vi "GEA3 HEWH Mixing Valve ERD List.vi"(8 "error in (no error)":errorcluster, 11 "Enable Electronic Mixing Valve (EMV) List":bool) -> (0 "error out":errorcluster, 2 "Headers":string[](array[string]), 3 "Read ERD List":T1[](array[typedef]) {"ERD Number" format="%.0x"})   [LabVIEW 2020]
uses:
  type defs/ERD Read Data In.ctl
  type defs/Data Type.ctl
  <vilib>/Utility/error.llb/whitespace.ctl
  library/GEA2_Toolkit.lvlib
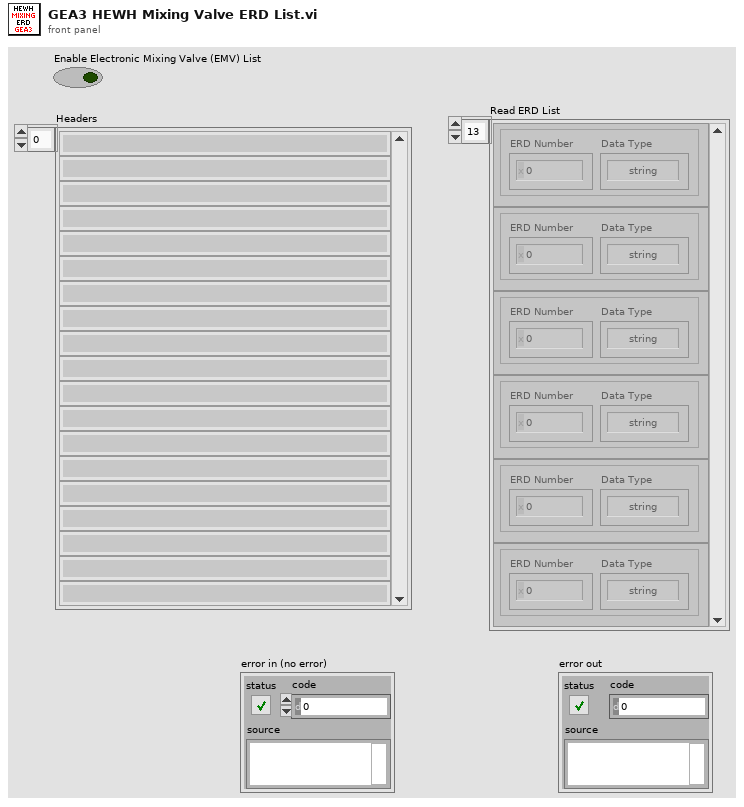
[diagram p1: front panel]
types:
  T1 = typedef "GEA2_Toolkit.lvlib/ERD Read Data In.ctl" = cluster{"ERD Number":u16, "Data Type":T2}
  T2 = typedef "GEA2_Toolkit.lvlib/Data Type.ctl" = enum16{"string", "boolean", "uint8_t", "uint16_t", "uint32_t", "uint64_t", "int8_t", "int16_t", "int32_t", "int64_t"}
  T3 = typedef "whitespace.ctl" = u16
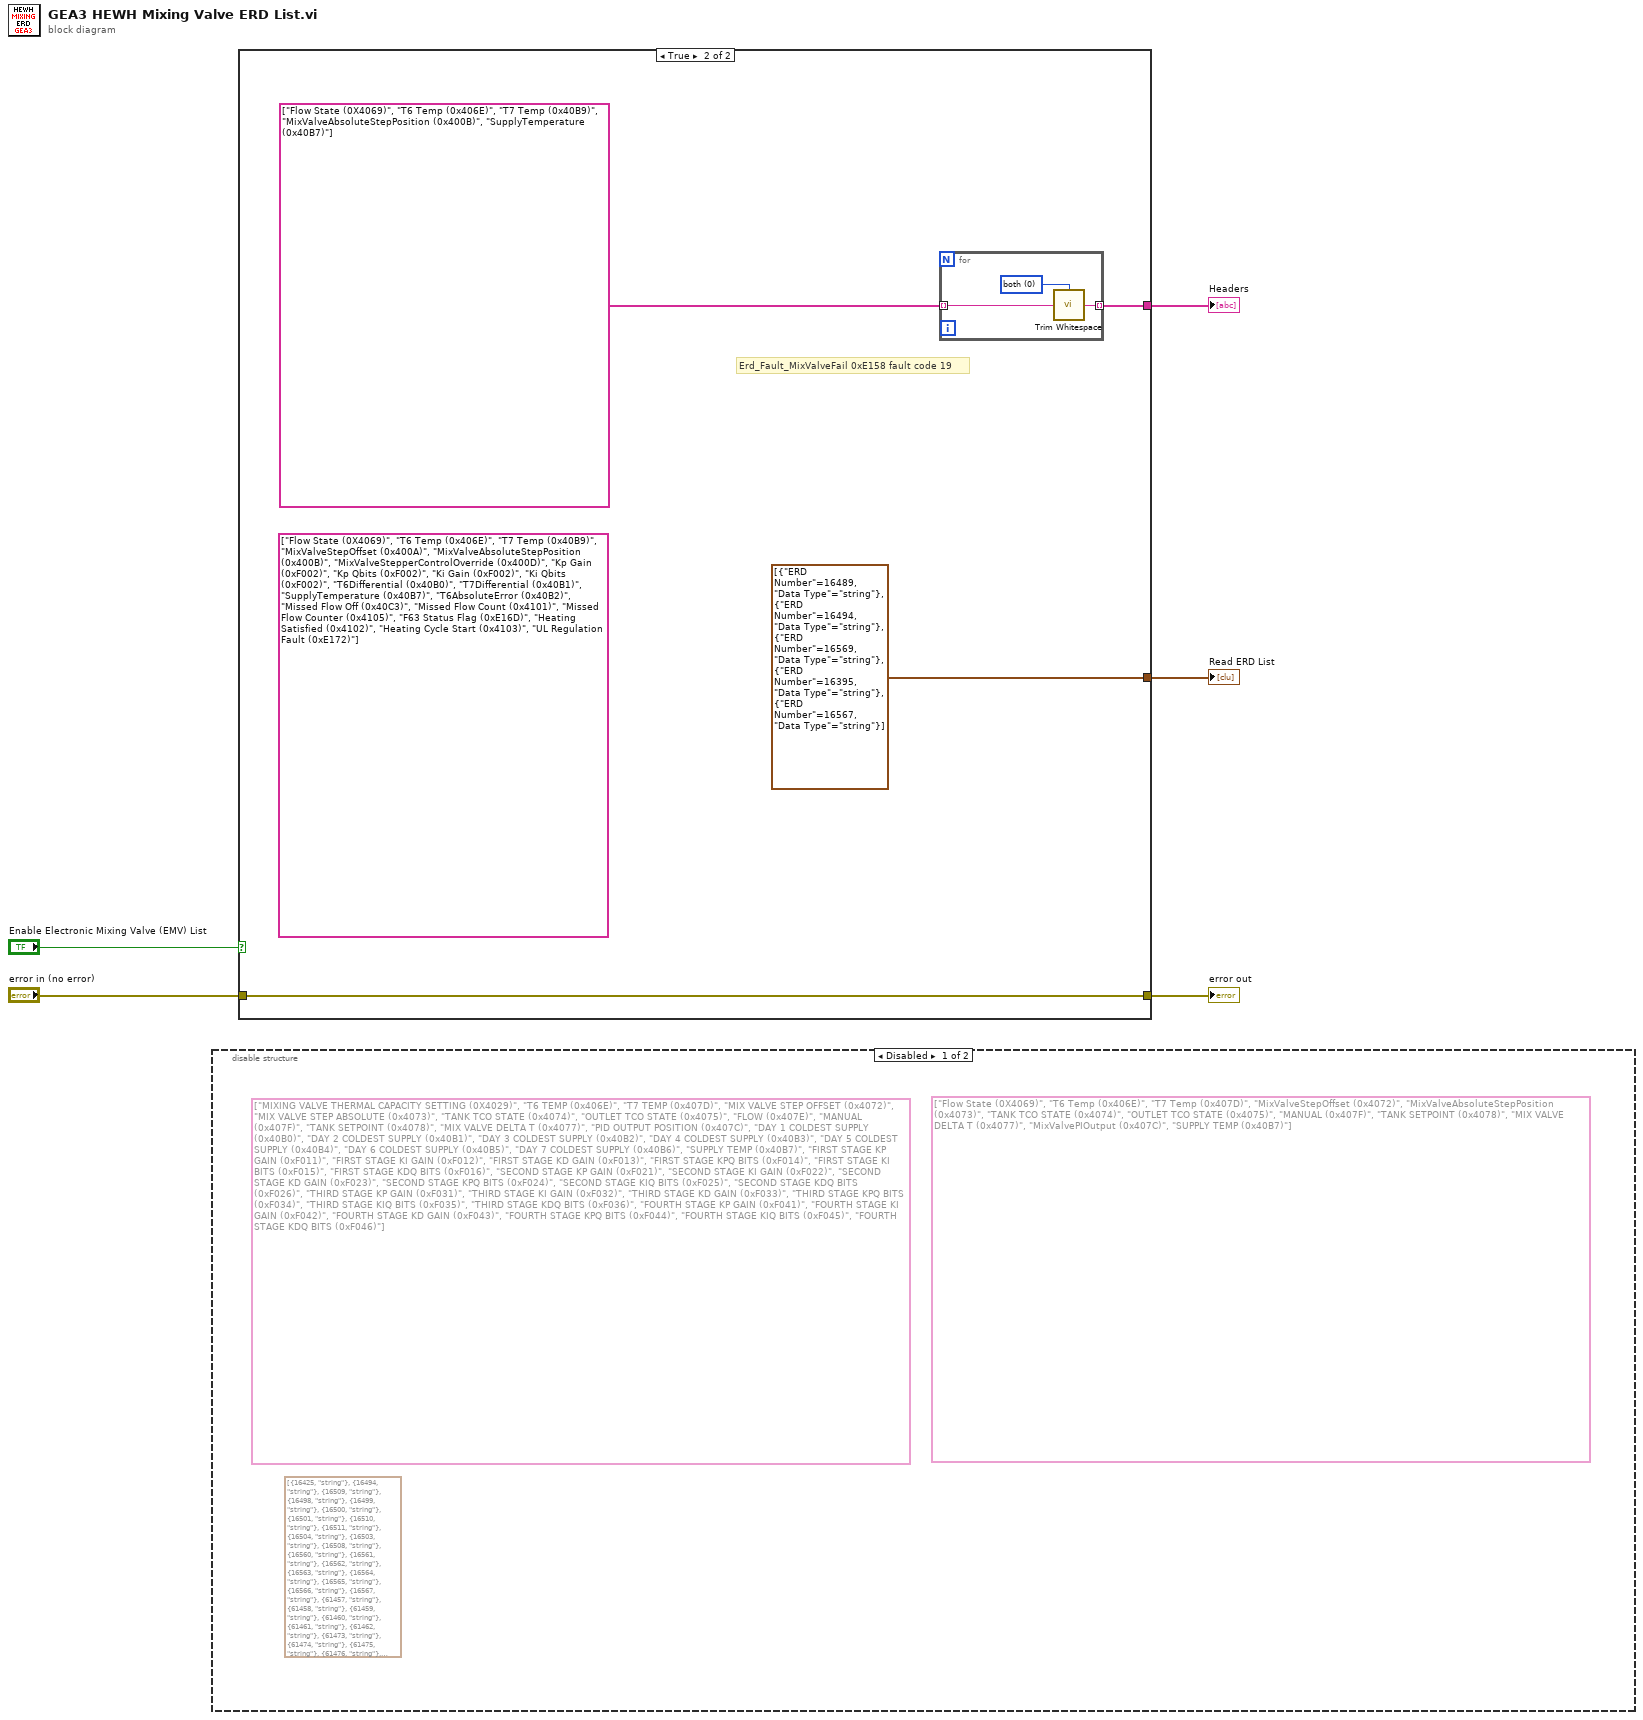
[diagram p0: block diagram]
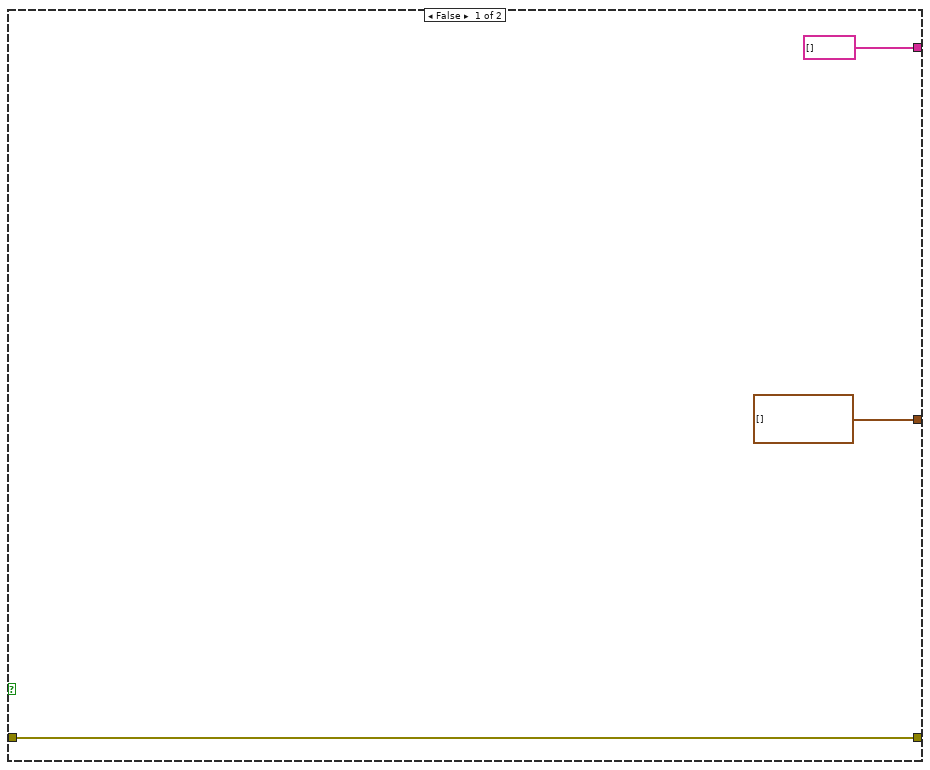
[diagram p3: hidden frame]
diagram:
  n1 = disable-structure shown="Disabled" {
    frame Disabled {
      (unwired) string[] ["Flow State (0X4069)", "T6 Temp (0x406E)", "T7 Temp (0x407D)", "MixValveStepOffset (0x4072)", "MixValveAbsoluteStepPosition (0x4073)", "TANK TCO STATE (0x4074)", "OUTLET TCO STATE (0x4075)", "MANUAL (0x407F)", "TANK SETPOINT (0x4078)", "MIX VALVE DELTA T (0x4077)", "MixValvePIOutput (0x407C)", "SUPPLY TEMP (0x40B7)"]
      (unwired) T1[] [{"ERD Number"=16425, "Data Type"=enum."string"}, {"ERD Number"=16494, "Data Type"=enum."string"}, {"ERD Number"=16509, "Data Type"=enum."string"}, {"ERD Number"=16498, "Data Type"=enum."string"}, {"ERD Number"=16499, "Data Type"=enum."string"}, {"ERD Number"=16500, "Data Type"=enum."string"}, {"ERD Number"=16501, "Data Type"=enum."string"}, {"ERD Number"=16510, "Data Type"=enum."string"}, {"ERD Number"=16511, "Data Type"=enum."string"}, {"ERD Number"=16504, "Data Type"=enum."string"}, {"ERD Number"=16503, "Data Type"=enum."string"}, {"ERD Number"=16508, "Data Type"=enum."string"}, {"ERD Number"=16560, "Data Type"=enum."string"}, {"ERD Number"=16561, "Data Type"=enum."string"}, {"ERD Number"=16562, "Data Type"=enum."string"}, {"ERD Number"=16563, "Data Type"=enum."string"}, {"ERD Number"=16564, "Data Type"=enum."string"}, {"ERD Number"=16565, "Data Type"=enum."string"}, {"ERD Number"=16566, "Data Type"=enum."string"}, {"ERD Number"=16567, "Data Type"=enum."string"}, {"ERD Number"=61457, "Data Type"=enum."string"}, {"ERD Number"=61458, "Data Type"=enum."string"}, {"ERD Number"=61459, "Data Type"=enum."string"}, {"ERD Number"=61460, "Data Type"=enum."string"}, {"ERD Number"=61461, "Data Type"=enum."string"}, {"ERD Number"=61462, "Data Type"=enum."string"}, {"ERD Number"=61473, "Data Type"=enum."string"}, {"ERD Number"=61474, "Data Type"=enum."string"}, {"ERD Number"=61475, "Data Type"=enum."string"}, {"ERD Number"=61476, "Data Type"=enum."string"}, {"ERD Number"=61477, "Data Type"=enum."string"}, {"ERD Number"=61478, "Data Type"=enum."string"}, {"ERD Number"=61489, "Data Type"=enum."string"}, {"ERD Number"=61490, "Data Type"=enum."string"}, {"ERD Number"=61491, "Data Type"=enum."string"}, {"ERD Number"=61492, "Data Type"=enum."string"}, {"ERD Number"=61493, "Data Type"=enum."string"}, {"ERD Number"=61494, "Data Type"=enum."string"}, {"ERD Number"=61505, "Data Type"=enum."string"}, {"ERD Number"=61506, "Data Type"=enum."string"}, {"ERD Number"=61507, "Data Type"=enum."string"}, {"ERD Number"=61508, "Data Type"=enum."string"}, {"ERD Number"=61509, "Data Type"=enum."string"}, {"ERD Number"=61510, "Data Type"=enum."string"}] ("Read ERD List")
      (unwired) string[] ["MIXING VALVE THERMAL CAPACITY SETTING (0X4029)", "T6 TEMP (0x406E)", "T7 TEMP (0x407D)", "MIX VALVE STEP OFFSET (0x4072)", "MIX VALVE STEP ABSOLUTE (0x4073)", "TANK TCO STATE (0x4074)", "OUTLET TCO STATE (0x4075)", "FLOW (0x407E)", "MANUAL (0x407F)", "TANK SETPOINT (0x4078)", "MIX VALVE DELTA T (0x4077)", "PID OUTPUT POSITION (0x407C)", "DAY 1 COLDEST SUPPLY (0x40B0)", "DAY 2 COLDEST SUPPLY (0x40B1)", "DAY 3 COLDEST SUPPLY (0x40B2)", "DAY 4 COLDEST SUPPLY (0x40B3)", "DAY 5 COLDEST SUPPLY (0x40B4)", "DAY 6 COLDEST SUPPLY (0x40B5)", "DAY 7 COLDEST SUPPLY (0x40B6)", "SUPPLY TEMP (0x40B7)", "FIRST STAGE KP GAIN (0xF011)", "FIRST STAGE KI GAIN (0xF012)", "FIRST STAGE KD GAIN (0xF013)", "FIRST STAGE KPQ BITS (0xF014)", "FIRST STAGE KI BITS (0xF015)", "FIRST STAGE KDQ BITS (0xF016)", "SECOND STAGE KP GAIN (0xF021)", "SECOND STAGE KI GAIN (0xF022)", "SECOND STAGE KD GAIN (0xF023)", "SECOND STAGE KPQ BITS (0xF024)", "SECOND STAGE KIQ BITS (0xF025)", "SECOND STAGE KDQ BITS (0xF026)", "THIRD STAGE KP GAIN (0xF031)", "THIRD STAGE KI GAIN (0xF032)", "THIRD STAGE KD GAIN (0xF033)", "THIRD STAGE KPQ BITS (0xF034)", "THIRD STAGE KIQ BITS (0xF035)", "THIRD STAGE KDQ BITS (0xF036)", "FOURTH STAGE KP GAIN (0xF041)", "FOURTH STAGE KI GAIN (0xF042)", "FOURTH STAGE KD GAIN (0xF043)", "FOURTH STAGE KPQ BITS (0xF044)", "FOURTH STAGE KIQ BITS (0xF045)", "FOURTH STAGE KDQ BITS (0xF046)"]
    }
    frame Enabled {
    }
  }
  n2 = case shown="True" "Enable Electronic Mixing Valve (EMV) List" {
    tunnel: [T1[] [] ("Read ERD List") T1[] [{"ERD Number"=16489, "Data Type"=enum."string"}, {"ERD Number"=16494, "Data Type"=enum."string"}, {"ERD Number"=16569, "Data Type"=enum."string"}, {"ERD Number"=16395, "Data Type"=enum."string"}, {"ERD Number"=16567, "Data Type"=enum."string"}] ("Read ERD List")] -> w5
    tunnel: "error in (no error)" -> [w8 w11]
    tunnel: [w8 w11] -> w3
    tunnel: [string[] [] ("array") w10] -> w1
    frame False {
    }
    frame True {
      (unwired) string[] ["Flow State (0X4069)", "T6 Temp (0x406E)", "T7 Temp (0x40B9)", "MixValveStepOffset (0x400A)", "MixValveAbsoluteStepPosition (0x400B)", "MixValveStepperControlOverride (0x400D)", "Kp Gain (0xF002)", "Kp Qbits (0xF002)", "Ki Gain (0xF002)", "Ki Qbits (0xF002)", "T6Differential (0x40B0)", "T7Differential (0x40B1)", "SupplyTemperature (0x40B7)", "T6AbsoluteError (0x40B2)", "Missed Flow Off (0x40C3)", "Missed Flow Count (0x4101)", "Missed Flow Counter (0x4105)", "F63 Status Flag (0xE16D)", "Heating Satisfied (0x4102)", "Heating Cycle Start (0x4103)", "UL Regulation Fault (0xE172)"]
      # "Erd_Fault_MixValveFail 0xE158 fault code 19"
      n3 = for {
        tunnel: string[] ["Flow State (0X4069)", "T6 Temp (0x406E)", "T7 Temp (0x40B9)", "MixValveAbsoluteStepPosition (0x400B)", "SupplyTemperature (0x40B7)"] -> [w14] mode=indexing
        tunnel: [w13] -> w10 mode=indexing
        w15 = T3 0 items=["both", "start of string", "end of string"] ("location (both)")
        n4 = call <vilib>:"Trim Whitespace.vi"("string"=w14, "location (both)"=w15) -> ("trimmed string"=w13:string)
      }
    }
  }
  "Read ERD List" <- w5
  "Headers" <- w1
  "error out" <- w3
